vi "Dialog box.vi"() -> ()   [LabVIEW 2020]
panel:
  in  "INPUT":string
  out "true":bool
  in  "button name (\"OK\")":string
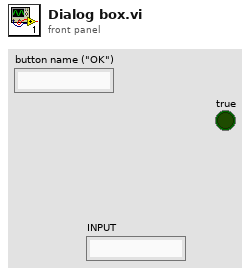
[diagram p1: front panel]
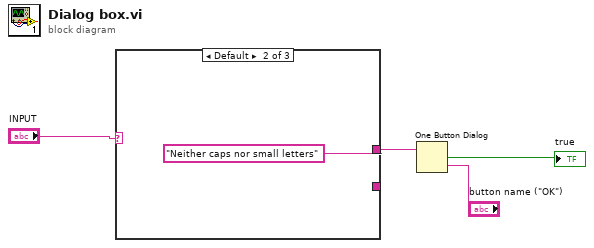
[diagram p0: block diagram]
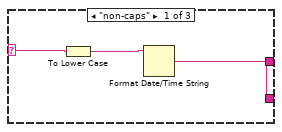
[diagram p2: hidden frame]
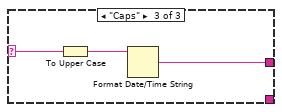
[diagram p3: hidden frame]
diagram:
  n1 = case shown="Default" "INPUT" {
    selector: "INPUT" -> [w6 _ w11]
    tunnel: [_ "Neither caps nor small letters" w9] -> w1
    tunnel: [w7 _ _] -> _
    frame "non-caps" {
      n2 = To Lower Case(string=w6) -> (all lower case string=w5:string)
      n3 = Format Date/Time String(time format string (%c)=w5) -> (date/time string=w7:string)  [unwired: 2 in]
    }
    frame Default {
    }
    frame "Caps" {
      n4 = To Upper Case(1:w11) -> (0:w10:string)
      n5 = Format Date/Time String(time format string (%c)=w10) -> (date/time string=w9:string)  [unwired: 2 in]
    }
  }
  n6 = One Button Dialog(message=w1, button name ("OK")="button name (\"OK\")") -> (true=→"true":bool)
